vi "Set Inline Buffer.vi"(8 "error in (no error)":errorcluster, 9 "size":u64, 10 "address":u64, 11 "Plugin Interface in":refnum<class "Plugin Interface.lvclass">) -> (0 "error out":errorcluster, 3 "Plugin Interface out":refnum<class "Plugin Interface.lvclass">)   [LabVIEW 2017, in "DSF Core.lvlib" / "Plugin Interface.lvclass"]
uses:
  Plugin Interface.lvclass
  C:/Users/Admin/Desktop/Data Sharing Framework/Source/Core/Engine/Classes/Interfaces/Interface/Interface.lvclass
  Command Data.ctl
  Command.ctl
  Command Parameters.ctl
  Interface/Interface.lvclass/Interface.ctl
  Response.ctl
  Write Plugin Command.vi
  Interface/Write Command.vi
  Interface/Write RT FIFO.vi
  Dispatcher/Command Timeout.vi
  Read Plugin Response.vi
  Dispatcher/Invalid Response Parameters.vi
  Dispatcher/Invalid Response.vi
  Interface/Interface.lvclass
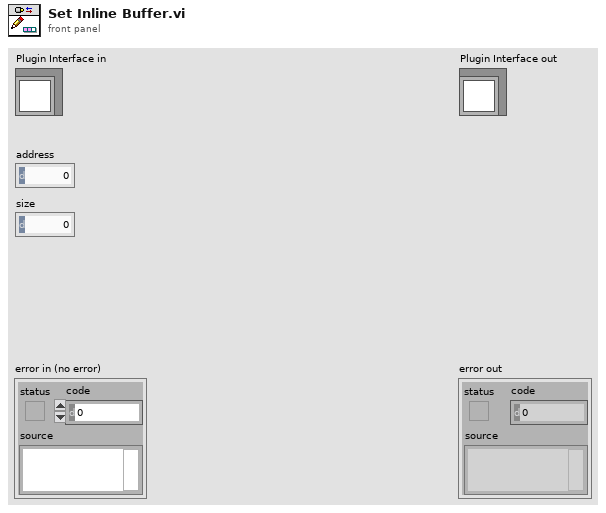
[diagram p1: front panel]
types:
  T1 = typedef "DSF Core.lvlib/Plugin Interface.lvclass/Command.ctl" = enum8{"Set Inline Buffer", "Rx", "Tx", "Shutdown"}
  T2 = typedef "DSF Core.lvlib/Plugin Interface.lvclass/Command Parameters.ctl" = cluster{"arg1":u64, "arg2":u64}
  T3 = typedef "DSF Core.lvlib/Plugin Interface.lvclass/Command Data.ctl" = cluster{"Command":T1, "Parameters":T2}
  T4 = typedef "DSF Core.lvlib/Plugin Interface.lvclass/Response Data.ctl" = cluster{"Response":T5, "Parameters":T6}
  T5 = typedef "DSF Core.lvlib/Plugin Interface.lvclass/Response.ctl" = enum8{"General Ack", "Shutting Down"}
  T6 = typedef "DSF Core.lvlib/Plugin Interface.lvclass/Response Parameters.ctl" = cluster{"arg1":u64, "arg2":u64}
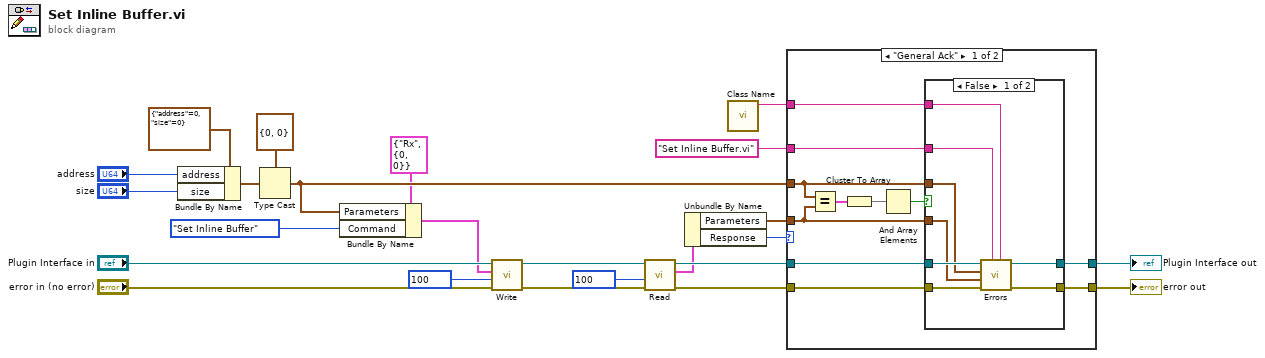
[diagram p0: block diagram]
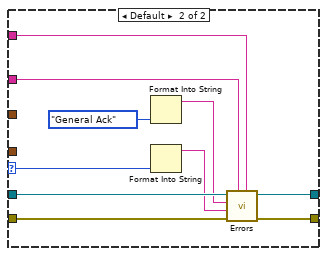
[diagram p3: hidden frame]
diagram:
  n1 = Bundle By Name(cluster=cluster{"address":u64, "size":u64} {"address"=0, "size"=0}, "address"="address", "size"="size") -> (w22:cluster{"address":u64, "size":u64})
  n2 = Type Cast(type=T2 {"arg1"=0, "arg2"=0} ("Command Parameters"), x=w22) -> (*(type *) &x=w4:T2)
  n3 = Bundle By Name(cluster=T3 {"Command"=enum."Rx", "Parameters"={"arg1"=0, "arg2"=0}} ("command"), "Parameters"=w4, "Command"=Command."Set Inline Buffer") -> (w15:T3)
  n4 = call-poly "Write.vi"("error in (no error)"="error in (no error)", "timeout in ms (0)"=100, "command"=w15, "Plugin Interface in"="Plugin Interface in") -> ("error out"=w13:errorcluster, "Plugin Interface out"=w14:refnum<class "Plugin Interface.lvclass">)  [unwired: 6 in]
  n5 = call-poly "Read.vi"("error in (no error)"=w13, "timeout in ms (0)"=100, "Plugin Interface in"=w14) -> ("error out"=w9:errorcluster, "response"=w7:T4, "Plugin Interface out"=w11:refnum<class "Plugin Interface.lvclass">)  [unwired: 5 in, 1 out]
  n6 = Unbundle By Name(w7) -> ("Parameters"=w5:T6, "Response"=w6:T5)
  n7 = call "Class Name.vi"() -> ("class name"=w1:string)  [unwired: 11 in]
  n8 = case shown="\"General Ack\"" w6 {
    selector: w6 -> [_ w49]
    tunnel: w11 -> [w35 w55]
    tunnel: [w33 w53] -> w10
    tunnel: w9 -> [w34 w54]
    tunnel: [w32 w52] -> w8
    tunnel: w5 -> [w25 _]
    tunnel: w4 -> [w26 _]
    tunnel: "Set Inline Buffer.vi" ("error source vi name") -> [w27 w51]
    tunnel: w1 -> [w28 w50]
    frame "General Ack" {
      n9 = Equal?(x=w26, y=w25) -> (x = y?=w31:cluster{"arg1":bool, "arg2":bool})
      n10 = Cluster To Array(cluster=w31) -> (array=w30:bool[])
      n11 = And Array Elements(Boolean array=w30) -> (logical AND=w29:bool)
      n12 = case shown="False" w29 {
        tunnel: w35 -> [w41 w45]
        tunnel: w34 -> [w43 w44]
        tunnel: [w40 w45] -> w33
        tunnel: [w42 w44] -> w32
        tunnel: w28 -> [w38 _]
        tunnel: w27 -> [w39 _]
        tunnel: w26 -> [w36 _]
        tunnel: w25 -> [w37 _]
        frame False {
          n13 = call-poly "Errors.vi"("error source class name"=w38, "error source vi name"=w39, "error in (no error)"=w43, "actual parameters"=w37, "expected parameters"=w36, "Interface in"=w41) -> ("error out"=w42:errorcluster, "Interface out"=w40:refnum<class "Plugin Interface.lvclass">)  [unwired: 4 in]
        }
        frame True {
          # "correct parameters"
        }
      }
    }
    frame Default {
      n14 = Format Into String(Response."General Ack" ("Response")) -> (resulting string=w46:string)  [unwired: 3 in, 1 out]
      n15 = Format Into String(w49) -> (resulting string=w48:string)  [unwired: 3 in, 1 out]
      n16 = call-poly "Errors.vi"("error source class name"=w50, "error source vi name"=w51, "error in (no error)"=w54, "actual response"=w48, "expected response"=w46, "Interface in"=w55) -> ("error out"=w52:errorcluster, "Interface out"=w53:refnum<class "Plugin Interface.lvclass">)  [unwired: 4 in]
    }
  }
  "error out" <- w8
  "Plugin Interface out" <- w10
